vi "Pref Group Name Const.vi"() -> (7 "Pref Group Name":string="IG_Protoc")   [LabVIEW 2020, in "LV-Protoc.lvlib" / "LV-Protoc.lvclass"]
uses:
  LV-Protoc.lvclass
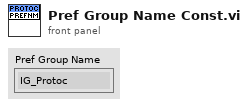
[diagram p1: front panel]
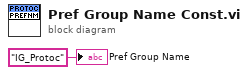
[diagram p0: block diagram]
diagram:
  "Pref Group Name" <- "IG_Protoc"
